vi "DtOLTimingSetInput.vi"(4 "Sync Mode":i32(ring) items=["None", "Master", "Slave"], 5 "Samples Per Channel":u32=1000, 6 "Num Buffers":u32=8, 7 "Sample Mode":enum16{"Finite Samples", "Continuous Samples"}(ring), 8 "error in (no error)":errorcluster, 9 "Timing":T1(ring), 10 "Sample Freq (Hz)":dbl=1000.0, 11 "Task in":i32) -> (0 "error out":errorcluster, 1 "Buffer Size":u32, 2 "Actual Sample Freq":dbl, 3 "Task out":i32)   [LabVIEW 2022 SP3]
doc: "Specifies all of the timing and buffer related details when streaming input data."
uses:
  DtLvLink.lvlib
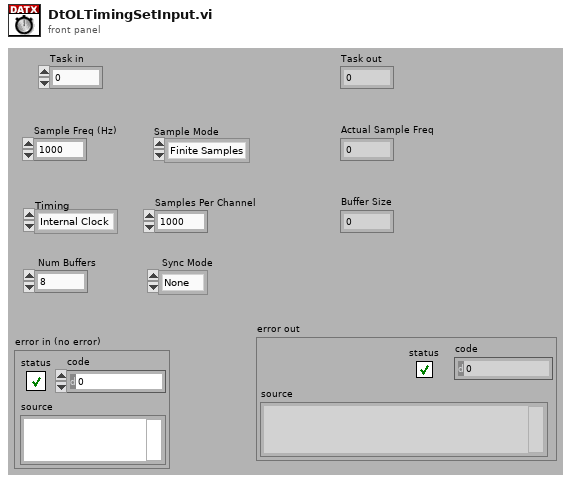
[diagram p1: front panel]
types:
  T1 = enum32{"Internal Clock", "External Clock", "No Timing"}
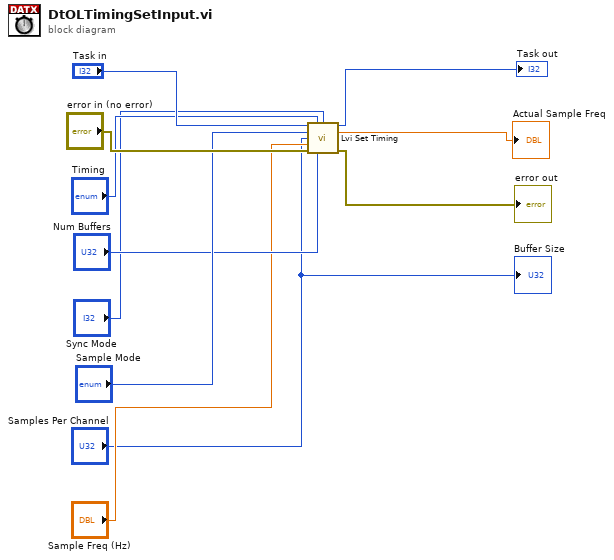
[diagram p0: block diagram]
diagram:
  n1 = call "Lvi Set Timing.vi"("TaskRef"="Task in", "ClkSource"="Timing", "SyncMode"="Sync Mode", "SampleMode"="Sample Mode", "PointsPerChan"="Samples Per Channel", "SampleRate"="Sample Freq (Hz)", "error in (no error)"="error in (no error)", "NumBuffers"="Num Buffers") -> ("TaskRef out"=→"Task out":i32, "ActualSampleRate"=→"Actual Sample Freq":dbl, "error out"=→"error out":errorcluster)  [unwired: 4 in, 1 out]
  "Buffer Size" <- "Samples Per Channel"
